vi "DefaultPsRole.vi"(9 "Game in":refnum<class "Game.lvclass">, 10 "DefaultPsRole in":refnum<class "DefaultPsRole.lvclass">) -> (2 "Robot out":refnum<class "Robot.lvclass">, 3 "DefaultPsRole out":refnum<class "DefaultPsRole.lvclass">)   [LabVIEW 2018, in "DefaultPsRole.lvclass"]
uses:
  DefaultPsRole.lvclass
  Robot_class/Robot.lvclass
  Game_class/Game.lvclass
  C:/Users/anton/Desktop/roboime/PS 2020.1/SSL_AI/Role_class/Role.lvclass
  Role_class/Role.lvclass/Role.ctl
  Role_class/Read Tacticbook.vi
  Role_class/Read tactic_index.vi
  Role_class/Write Tacticbook.vi
  Role_class/Write tactic_index.vi
  Role_class/Read RobotRef.vi
  Tacticbook_class/Tacticbook.lvclass
  DefaultPsTactic_class/DefaultPsTactic.lvclass
panel:
  out "Game out":refnum<class "Game.lvclass">
  out "error out 2":errorcluster
  in  "error in (no error) 2":errorcluster
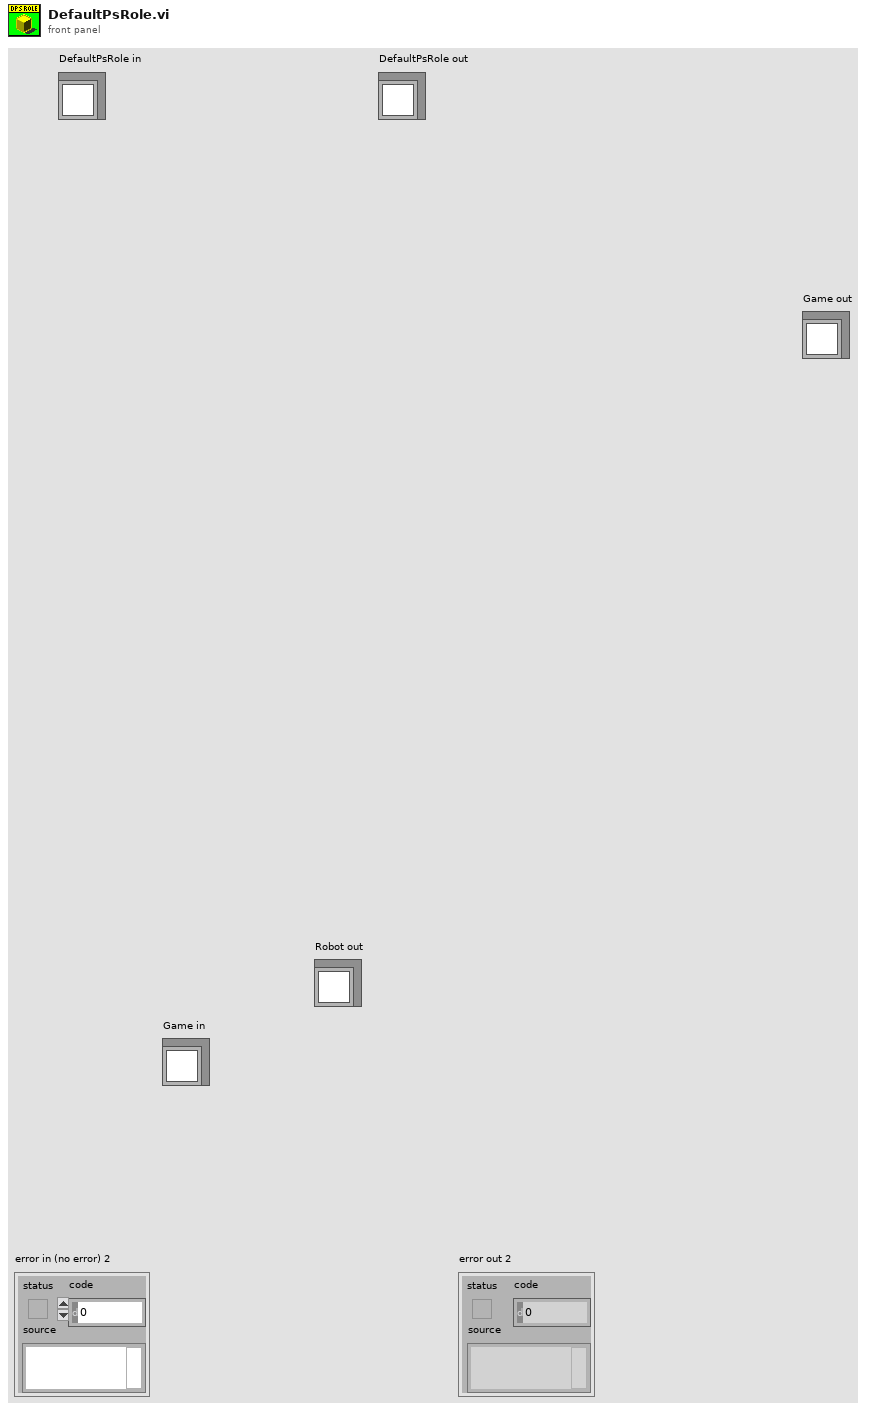
[diagram p1: front panel]
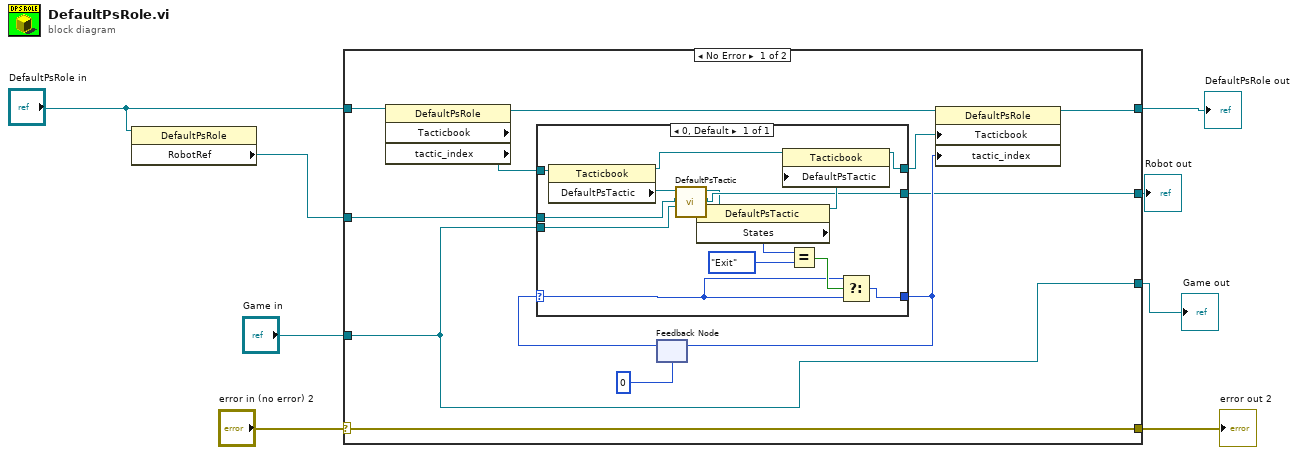
[diagram p0: block diagram]
diagram:
  n1 = property class="DefaultPsRole"(reference="DefaultPsRole in") -> ("RobotRef"=w4:refnum<class "Robot.lvclass">)  [unwired: 1 in, 2 out]
  n2 = case shown="No Error" "error in (no error) 2" {
    selector: "error in (no error) 2" -> [w20 w38]
    tunnel: [w20 w38] -> w7
    tunnel: [w18 w37] -> w3
    tunnel: "DefaultPsRole in" -> [w19 w37]
    tunnel: w4 -> [w12 w36]
    tunnel: [w11 w36] -> w6
    tunnel: [w9 w35] -> w1
    tunnel: "Game in" -> [w9 w35]
    frame No Error {
      n3 = property class="DefaultPsRole" props=["Tacticbook", "tactic_index"](reference=w19) -> (reference out=w17:refnum<class "DefaultPsRole.lvclass">, "Tacticbook"=w14:refnum<class "Tacticbook.lvclass">)  [unwired: 1 in, 2 out]
      n4 = feedback #1(0) -> (w15:i32)
      n5 = case shown="0, Default" w15 {
        selector: w15 -> [w21]
        tunnel: [w31] -> w13
        tunnel: w14 -> [w34]
        tunnel: w12 -> [w26]
        tunnel: [w24] -> w11
        tunnel: [w28] -> w10
        tunnel: w9 -> [w25]
        frame 0, Default {
          n6 = property class="Tacticbook"(reference=w34) -> (reference out=w30:refnum<class "Tacticbook.lvclass">, "DefaultPsTactic"=w27:refnum<class "DefaultPsTactic.lvclass">)  [unwired: 1 in, 1 out]
          n7 = call "DefaultPsTactic.vi"("Game in"=w25, "Robot"=w26, "DefaultPsTactic in"=w27) -> ("Robot out"=w24:refnum<class "Robot.lvclass">, "DefaultPsTactic out"=w23:refnum<class "DefaultPsTactic.lvclass">)  [unwired: 7 in]
          n8 = property class="DefaultPsTactic"(reference=w23) -> (reference out=w29:refnum<class "DefaultPsTactic.lvclass">, "States"=w33:enum16{"Exit", "AttackPs", "DefensePs"})  [unwired: 1 in, 1 out]
          n9 = property class="Tacticbook"(reference=w30, "DefaultPsTactic"=w29) -> (reference out=w28:refnum<class "Tacticbook.lvclass">)  [unwired: 1 in, 1 out]
          n10 = Equal?(x=w33, y=enum16{"Exit", "AttackPs", "DefensePs"}."Exit" ("States")) -> (x = y?=w32:bool)
          n11 = Select(t=w21, s=w32, f=w21) -> (s? t:f=w31:i32)
        }
      }
      n12 = feedback-in #1(w13) -> ()
      n13 = property class="DefaultPsRole"(reference=w17, "Tacticbook"=w10, "tactic_index"=w13) -> (reference out=w18:refnum<class "DefaultPsRole.lvclass">)  [unwired: 1 in, 1 out]
    }
    frame Error {
    }
  }
  "error out 2" <- w7
  "Robot out" <- w6
  "DefaultPsRole out" <- w3
  "Game out" <- w1
